vi "Gamepad Test App.vi"() -> ()   [LabVIEW 2011, in "LVH-PS4.lvlib"]
uses:
  LVH-PS4.lvlib
  Private/Type Defs/Indicators/Controller.ctl
  Private/Type Defs/Indicators/Square.ctl
  Private/Type Defs/Indicators/X.ctl
  Private/Type Defs/Indicators/Circle.ctl
  Private/Type Defs/Indicators/Triangle.ctl
  Private/Type Defs/Indicators/L1.ctl
  Private/Type Defs/Indicators/R1.ctl
  Private/Type Defs/Indicators/Share.ctl
  Private/Type Defs/Indicators/Options.ctl
  Private/Type Defs/Indicators/PS.ctl
  Private/Type Defs/Indicators/Pad_Button.ctl
  Private/Type Defs/Indicators/Dpad.ctl
  Private/Type Defs/Indicators/Slider.ctl
  <vilib>/Utility/inputDevices.llb/closeJoystick.vi
  <vilib>/Utility/inputDevices.llb/joystickAcquire.vi
panel:
  out "PS4 Controller":T1={"Square Button"=FALSE, "X Button"=FALSE, "Circle Button"=FALSE, "Triangle Button"=FALSE, "L1"=FALSE, "R1"=FALSE, "Share Button"=FALSE, "Options Button"=FALSE, "PS Button"=FALSE, "Pad Button"=FALSE, "D-Pad"=5, "L2"=0, "R2"=0, "Thumbstick_Left"={[], []}, "Thumbstick_Right"={[], []}} {"R2" scale=-32768.0..32767.0; "L2" scale=-32768.0..32767.0}
  out "direction info":T14
  out "button info":T15
  out "axis info":T16
  out "joystick info":T17(array[cluster])
  in  "Stop Button":bool
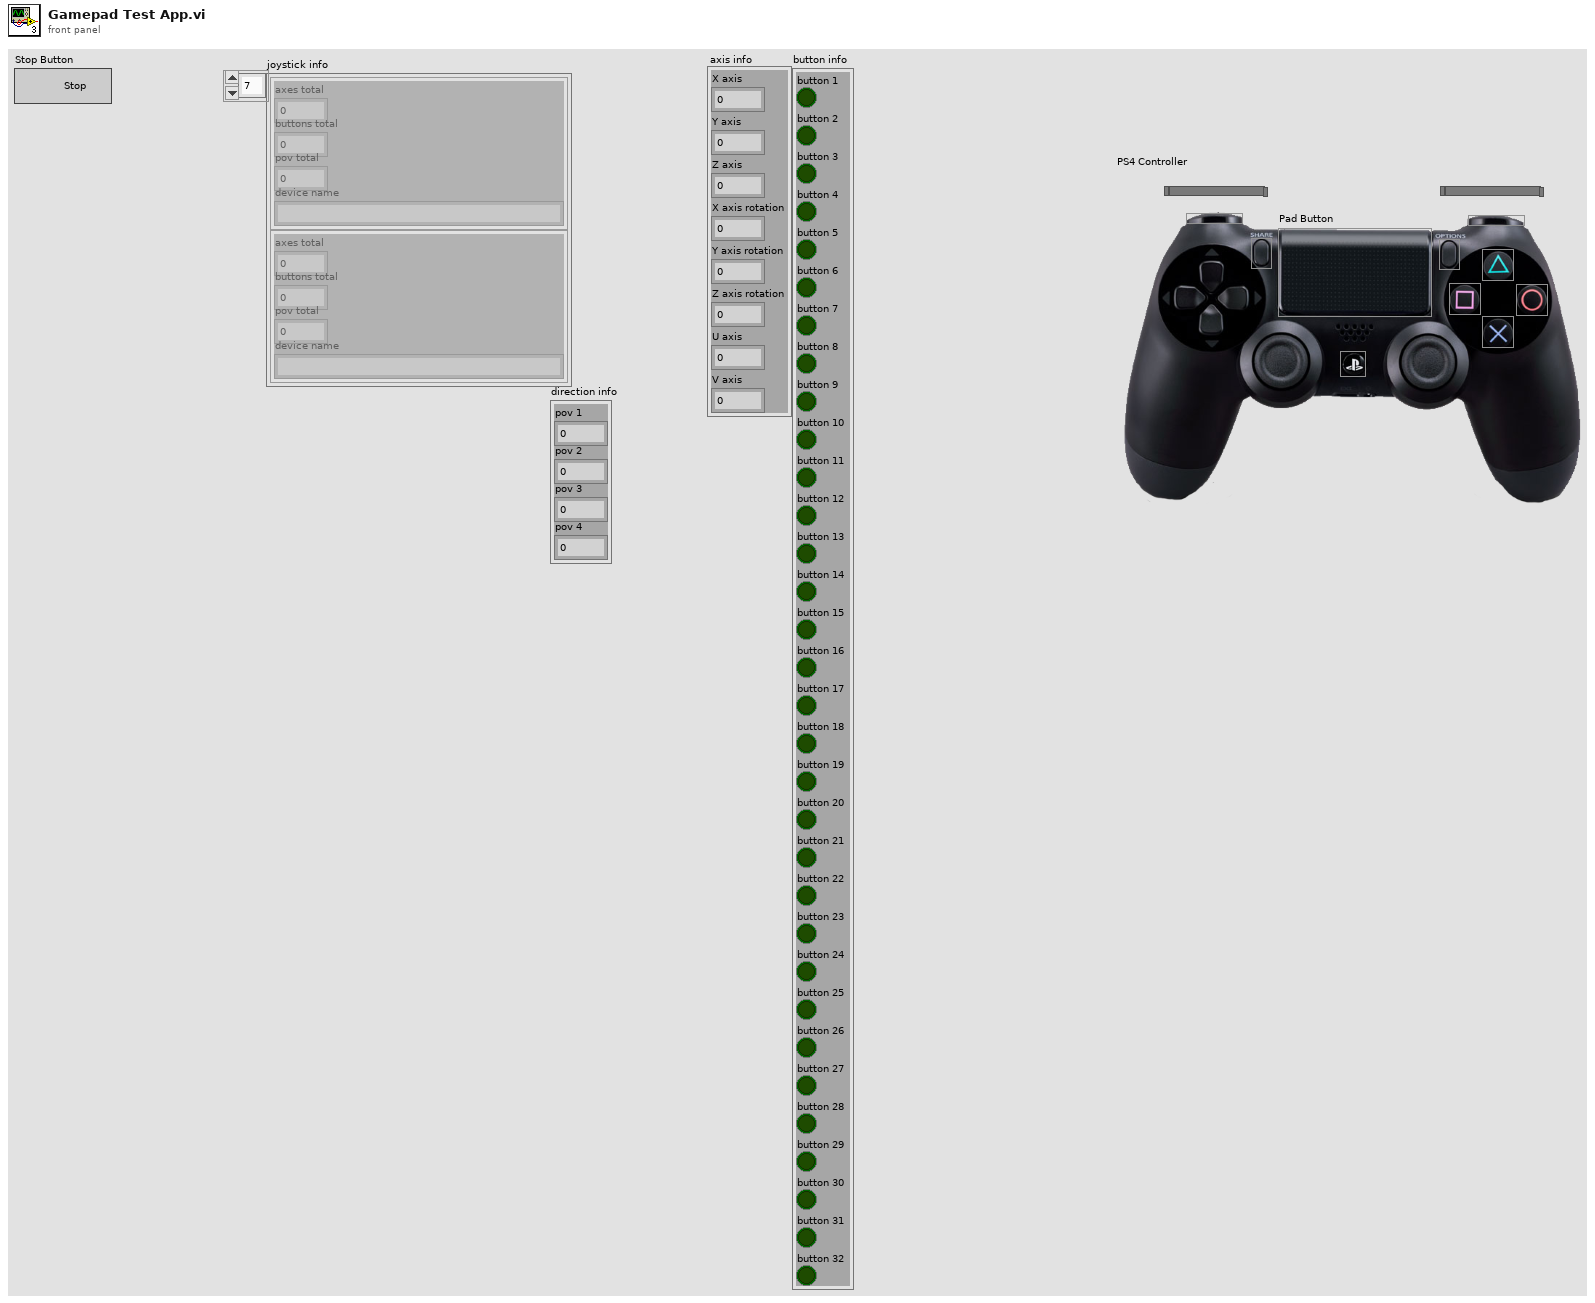
[diagram p1: front panel]
types:
  T1 = typedef "LVH-PS4.lvlib/Controller.ctl" = cluster{"Square Button":T2, "X Button":T3, "Circle Button":T4, "Triangle Button":T5, "L1":T6, "R1":T7, "Share Button":T8, "Options Button":T9, "PS Button":T10, "Pad Button":T11, "D-Pad":T12, "L2":T13, "R2":T13, "Thumbstick_Left":cluster{i32[], i32[]}, "Thumbstick_Right":cluster{i32[], i32[]}}
  T2 = typedef "LVH-PS4.lvlib/Square.ctl" = bool
  T3 = typedef "LVH-PS4.lvlib/X.ctl" = bool
  T4 = typedef "LVH-PS4.lvlib/Circle.ctl" = bool
  T5 = typedef "LVH-PS4.lvlib/Triangle.ctl" = bool
  T6 = typedef "LVH-PS4.lvlib/L1.ctl" = bool
  T7 = typedef "LVH-PS4.lvlib/R1.ctl" = bool
  T8 = typedef "LVH-PS4.lvlib/Share.ctl" = bool
  T9 = typedef "LVH-PS4.lvlib/Options.ctl" = bool
  T10 = typedef "LVH-PS4.lvlib/PS.ctl" = bool
  T11 = typedef "LVH-PS4.lvlib/Pad_Button.ctl" = bool
  T12 = typedef "LVH-PS4.lvlib/Dpad.ctl" = u16
  T13 = typedef "LVH-PS4.lvlib/Slider.ctl" = i32
  T14 = cluster{"pov 1":i32, "pov 2":i32, "pov 3":i32, "pov 4":i32}
  T15 = cluster{"button 1":bool, "button 2":bool, "button 3":bool, "button 4":bool, "button 5":bool, "button 6":bool, "button 7":bool, "button 8":bool, "button 9":bool, "button 10":bool, "button 11":bool, "button 12":bool, "button 13":bool, "button 14":bool, "button 15":bool, "button 16":bool, "button 17":bool, "button 18":bool, "button 19":bool, "button 20":bool, "button 21":bool, "button 22":bool, "button 23":bool, "button 24":bool, "button 25":bool, "button 26":bool, "button 27":bool, "button 28":bool, "button 29":bool, "button 30":bool, "button 31":bool, "button 32":bool}
  T16 = cluster{"X axis":i32, "Y axis":i32, "Z axis":i32, "X axis rotation":i32, "Y axis rotation":i32, "Z axis rotation":i32, "U axis":i32, "V axis":i32}
  T17 = cluster{"axes total":u32, "buttons total":u32, "pov total":u32, "device name":string}[]
  T18 = typedef "LVH-Xbox-One-Controller.lvlib/DPad Enum.ctl" = enum16{"Idle", "Up", "Up / Right", "Right", "Down / Right", "Down", "Down / Left", "Left", "Up / Left"}
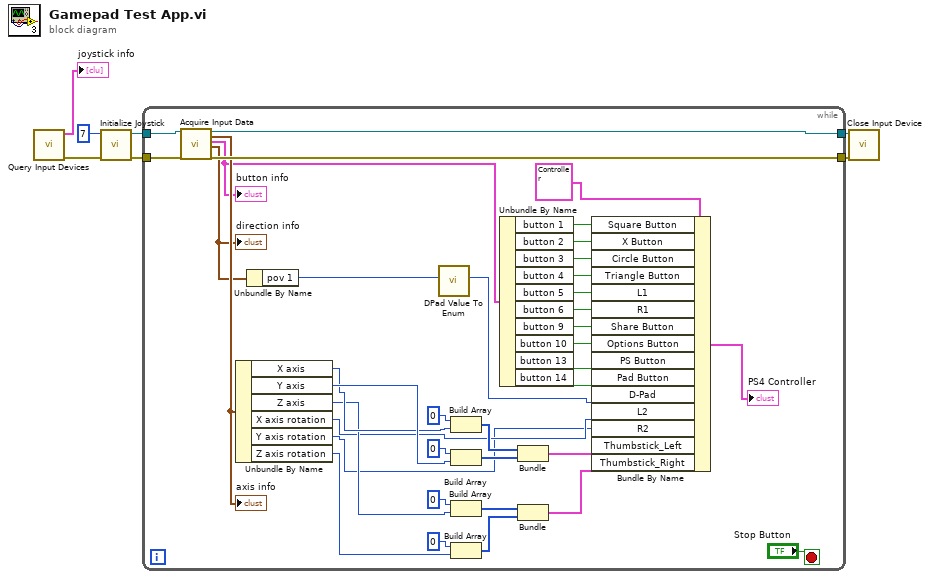
[diagram p0: block diagram]
diagram:
  n1 = call <vilib>:"Query Input Devices.vi"() -> ("error out"=w7:errorcluster, "joystick info"=→"joystick info":T17)  [unwired: 8 in, 2 out]
  n2 = call <vilib>:"Initialize Joystick.vi"("error in (no error)"=w7, "device index"=7) -> ("error out"=w6:errorcluster, "device ID"=w3:refnum<k1>)  [unwired: 8 in]
  n3 = while {
    tunnel: w6 -> [w44]
    tunnel: [w43] -> w5
    tunnel: [w42] -> w4
    tunnel: w3 -> [w41]
    stop <- "Stop Button" stop-if-true
    n4 = call-poly <vilib>:"Acquire Input Data.vi"("device ID"=w41, "error in (no error)"=w44) -> ("device ID"=w42:refnum<k1>, "axis info"=w40:T16, "button info"=w25:T15, "direction info"=w14:T14, "error out"=w43:errorcluster)  [unwired: 13 in]
    "axis info" <- w40
    "button info" <- w25
    "direction info" <- w14
    n5 = Unbundle By Name(w40) -> ("X axis"=w36:i32, "Y axis"=w39:i32, "Z axis"=w11:i32, "X axis rotation"=w9:i32, "Y axis rotation"=w8:i32, "Z axis rotation"=w27:i32)
    n6 = Unbundle By Name(w14) -> ("pov 1"=w13:i32)
    n7 = call "DPad Value To Enum.vi"("D-Pad Value"=w13) -> ("D-Pad Enum"=w12:T18)  [unwired: 10 in]
    n8 = Build Array(0 ("element"), w36) -> (w35:i32[])
    n9 = Build Array(0 ("element"), w39) -> (w34:i32[])
    n10 = Build Array(0 ("element"), w11) -> (w30:i32[])
    n11 = Build Array(0 ("element"), w27) -> (w31:i32[])
    n12 = Unbundle By Name(w25) -> ("button 1"=w24:bool, "button 2"=w23:bool, "button 3"=w22:bool, "button 4"=w21:bool, "button 5"=w20:bool, "button 6"=w19:bool, "button 9"=w18:bool, "button 10"=w17:bool, "button 13"=w16:bool, "button 14"=w15:bool)
    n13 = Bundle(w35, w34) -> (w32:cluster{i32[], i32[]})  [unwired: 1 in]
    n14 = Bundle(w30, w31) -> (w26:cluster{i32[], i32[]})  [unwired: 1 in]
    n15 = Bundle By Name(cluster=T1 {"Square Button"=FALSE, "X Button"=FALSE, "Circle Button"=FALSE, "Triangle Button"=FALSE, "L1"=FALSE, "R1"=FALSE, "Share Button"=FALSE, "Options Button"=FALSE, "PS Button"=FALSE, "Pad Button"=FALSE, "D-Pad"=5, "L2"=0, "R2"=0, "Thumbstick_Left"={[], []}, "Thumbstick_Right"={[], []}} ("PS4 Controller"), "Square Button"=w24, "X Button"=w23, "Circle Button"=w22, "Triangle Button"=w21, "L1"=w20, "R1"=w19, "Share Button"=w18, "Options Button"=w17, "PS Button"=w16, "Pad Button"=w15, "D-Pad"=w12, "L2"=w9, "R2"=w8, "Thumbstick_Left"=w32, "Thumbstick_Right"=w26) -> (→"PS4 Controller":T1)
  }
  n16 = call-poly <vilib>:"Close Input Device.vi"("error in (no error)"=w5, "device ID"=w4) -> ()  [unwired: 8 in, 1 out]
